vi "Evaluate Read Data By ID.vi"(1 "String In":string) -> (0 "Test OK":bool)   [LabVIEW 2022 SP3]
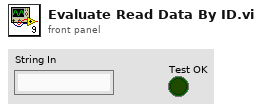
[diagram p1: front panel]
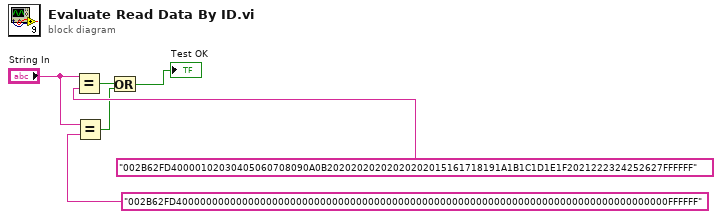
[diagram p0: block diagram]
diagram:
  n1 = Equal?(x="String In", y="002B62FD40000102030405060708090A0B20202020202020202015161718191A1B1C1D1E1F2021222324252627FFFFFF") -> (x = y?=w3:bool)
  n2 = Equal?(x="String In", y="002B62FD4000000000000000000000000000000000000000000000000000000000000000000000000000000000FFFFFF") -> (x = y?=w2:bool)
  n3 = Or(x=w3, y=w2) -> (x .or. y?=→"Test OK":bool)
